vi "Send data.vi"(8 "error in (no error)":T1, 10 "group":string, 11 "Data":refnum<class "mmWave data.lvclass">) -> (0 "error out":T1)   [LabVIEW 2019, in "Shared.lvlib"]
doc: "Trigger New data event:\n- group (tx or rx)\n- Data - object containing new IQ burst"
uses:
  Shared.lvlib
  mmWave data_class/mmWave data.lvclass
  Data message cluster.ctl
  Comm GV.vi
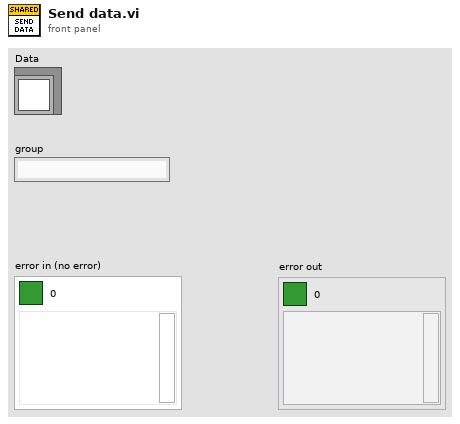
[diagram p1: front panel]
types:
  T1 = cluster{"Boolean Round":bool, "code":i32, "source":string}
  T2 = typedef "Shared.lvlib/Data message cluster.ctl" = cluster{"group  ":string, "Data":refnum<class "mmWave data.lvclass">}
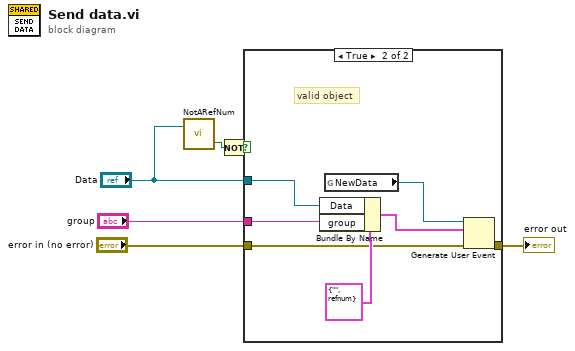
[diagram p0: block diagram]
diagram:
  n1 = call-dynamic "NotARefNum.vi"("reference in"="Data") -> ("not a refnum?"=w2:bool)  [unwired: 1 in, 1 out]
  n2 = Not(x=w2) -> (.not. x?=w1:bool)
  n3 = case shown="True" w1 {
    tunnel: [w7 w11] -> w6
    tunnel: "error in (no error)" -> [w7 w10]
    tunnel: "group" -> [_ w9]
    tunnel: "Data" -> [_ w8]
    frame False {
      # "invalid data, skip sending it"
    }
    frame True {
      # "valid object"
      n4 = Bundle By Name(cluster=T2 {"group  "="", "Data"=refnum} ("event data"), "Data"=w8, "group"=w9) -> (w13:T2)
      n5 = global read "Comm GV.vi" "NewData"() -> (w14:refnum<user-event>)
      n6 = Generate User Event(user event=w14, event data cluster=w13, error in=w10) -> (error out=w11:errorcluster)  [unwired: 1 in, 1 out]
    }
  }
  "error out" <- w6
